vi "Query Error Log.vi"(6 "timeout (ms)":i32=5000, 8 "error in":errorcluster, 10 "query_all":bool, 11 "gRPC ID in":T2) -> (0 "error out":errorcluster, 2 "error_info":T1[](array[typedef]), 3 "gRPC ID out":T2)   [LabVIEW 2021, in "CIFManagerClientWrapper.lvlib"]
uses:
  CIFManagerClientWrapper.lvlib
  <vilib>/gRPC/LabVIEW gRPC Library/Shared/grpcId.ctl
  CIF_Manager_client/RPC Messages/cif_manager_ErrorInfo.ctl
  CIF_Manager_client/RPC Messages/cif_manager_QueryErrorsRequest.ctl
  CIF_Manager_client/RPC Messages/cif_manager_QuerySettings.ctl
  CIF_Manager_client/CIF_Manager_client.lvlib
  <vilib>/gRPC/LabVIEW gRPC Library/grpc-lvsupport-release.lvlib
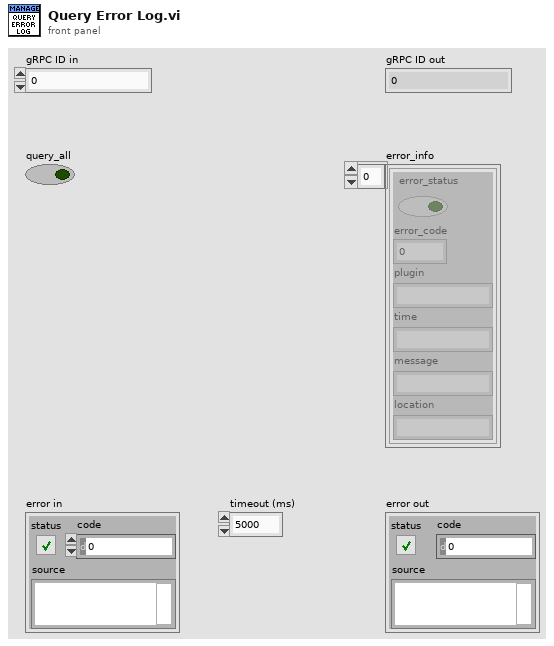
[diagram p1: front panel]
types:
  T1 = typedef "CIF_Manager_client.lvlib/cif_manager_ErrorInfo.ctl" = cluster{"error_status":bool, "error_code":i32, "plugin":string, "time":string, "message":string, "location":string}
  T2 = typedef "grpc-lvsupport-release.lvlib/grpcId.ctl" = u64
  T3 = typedef "CIF_Manager_client.lvlib/cif_manager_QueryErrorsRequest.ctl" = cluster{"query_settings":T4}
  T4 = typedef "CIF_Manager_client.lvlib/cif_manager_QuerySettings.ctl" = cluster{"query_all":bool}
  T5 = typedef "CIF_Manager_client.lvlib/cif_manager_QueryErrorsResponse.ctl" = cluster{"error_info_list":T6}
  T6 = typedef "CIF_Manager_client.lvlib/cif_manager_ErrorInfoList.ctl" = cluster{"error_info":T1[]}
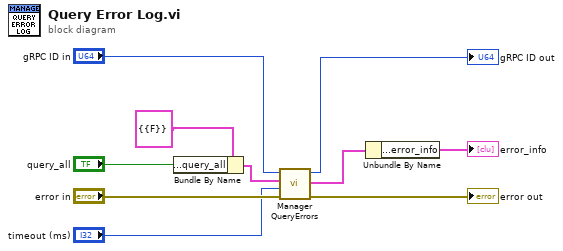
[diagram p0: block diagram]
diagram:
  n1 = Bundle By Name(cluster=T3 {"query_settings"={"query_all"=FALSE}} ("Request Data"), "query_settings.query_all"="query_all") -> (w2:T3)
  n2 = call "Manager QueryErrors.vi"("error in"="error in", "timeout (ms)"="timeout (ms)", "Request Data"=w2, "gRPC ID"="gRPC ID in") -> ("error out"=→"error out":errorcluster, "Response Data"=w5:T5, "gRPC ID out"=→"gRPC ID out":T2)  [unwired: 5 in]
  n3 = Unbundle By Name(w5) -> ("error_info_list.error_info"=→"error_info":T1[])
